vi "Send Emergency Stop.vi"(8 "error in (no error)":errorcluster, 11 "Message Enqueuer":refnum<class "Message Enqueuer.lvclass">) -> (0 "error out":errorcluster)   [LabVIEW 2020, in "Actor Framework.lvlib" / "Stop Msg.lvclass"]
doc: "<p>(<strong>Filename</strong>: <span class=\"dnl\">Actor Framework.lvlib:Stop Msg.lvclass:Send Emergency Stop.vi</span>)</p>\n\n<p>Sends an Emergency Stop message to an actor, triggering the actor to shut down as quickly as possible. This message has critical priority, meaning it will be processed before all messages that are already in the queue.</p>"
uses:
  Stop Msg.lvclass
  Message Enqueuer/Message Enqueuer.lvclass
  Stop Msg.lvclass/Stop Msg.ctl
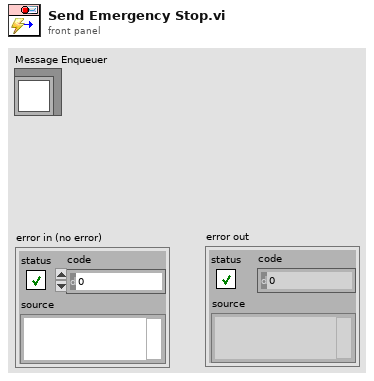
[diagram p1: front panel]
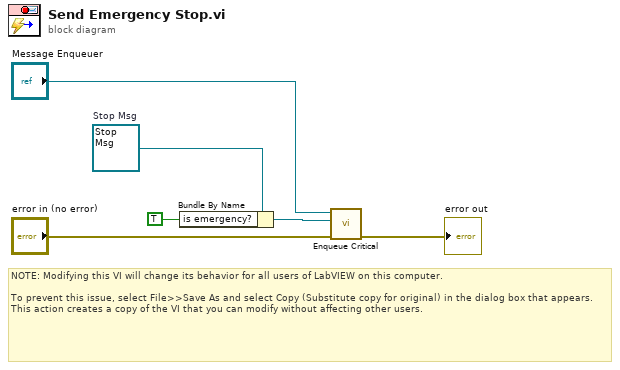
[diagram p0: block diagram]
diagram:
  w6 = refnum<class "Stop Msg.lvclass"> refnum  # Stop Msg
  # "NOTE: Modifying this VI will change its behavior for all users of LabVIEW on this computer.\n\nTo prevent this issue, select File>>Save As and select Copy (Substitute copy for original) in the dialog box that appears. This action creates a copy of the VI that you can modify without affecting other users."
  n1 = Bundle By Name(cluster=w6, "is emergency?"=TRUE) -> (w3:refnum<class "Stop Msg.lvclass">)
  n2 = call "Enqueue Critical.vi"("error in (no error)"="error in (no error)", "Message"=w3, "Message Enqueuer in"="Message Enqueuer") -> ("error out"=→"error out":errorcluster)  [unwired: 7 in, 1 out]
